vi "Cz.vi"(10 "C_reg":dbl, 11 "C":dbl) -> (3 "Cz":dbl)   [LabVIEW 2020]
doc: "SubVI wyznacza pojemność zastępczą połączonych kondensatorów w Q-metrze.\n\nDane wejściowe:\nC - pojemność badanego kondesatora\nC_reg - pojemność regulowana (ustawiona na Q-metrze)"
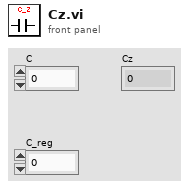
[diagram p1: front panel]
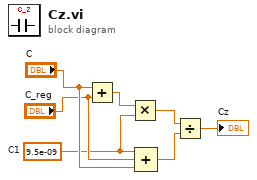
[diagram p0: block diagram]
diagram:
  w2 = 9.5e-09  # C1
  n1 = Add(x="C", y="C_reg") -> (x+y=w1:dbl)
  n2 = Multiply(x=w1, y=w2) -> (x*y=w5:dbl)
  n3 = Compound Arithmetic op=ADD(w2, "C_reg", "C") -> (w6:dbl)
  n4 = Divide(x=w5, y=w6) -> (x/y=→"Cz":dbl)
